vi "停止.vi"(1 "停止":bool) -> (0 "停止报文发送":string)   [LabVIEW 2023]
uses:
  <vilib>/Instr/_visa.llb/VISA Configure Serial Port (Instr).vi
panel:
  out "读取缓冲区":string
  out "返回数":u32
  in  "VISA resource name":refnum<visa-resource-name>="COM8" caption="VISA资源名称"
  out "错误输出":errorcluster
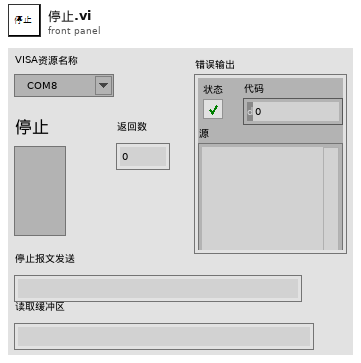
[diagram p1: front panel]
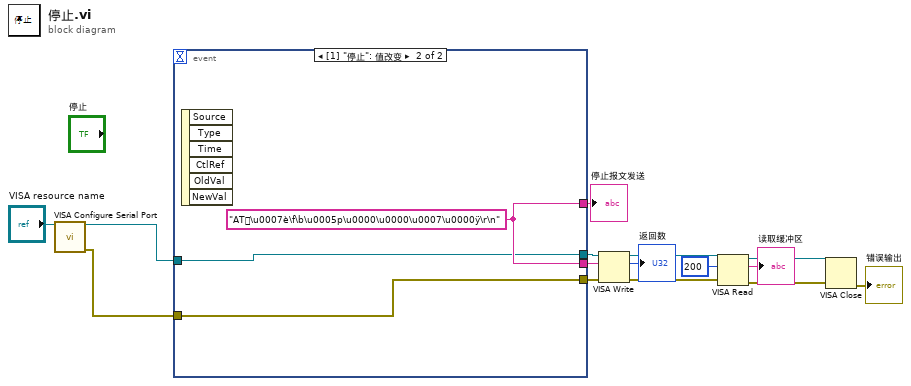
[diagram p0: block diagram]
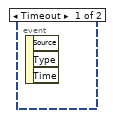
[diagram p2: hidden frame]
diagram:
  n1 = call-poly "VISA Configure Serial Port"("VISA resource name"="VISA resource name") -> ("VISA resource name out"=w6:refnum<visa-resource-name>, "error out"=w3:errorcluster)  [unwired: 13 in]
  n2 = event shown="[1] \"停止\": 值改变" {
    selector: _ -> [_ _]
    dyn-events: _ -> [_ _]
    timeout: _ -> [_ _]
    tunnel: [_ w18] -> w15
    tunnel: [_ w18] -> w7
    tunnel: w6 -> [_ w17]
    tunnel: [_ w17] -> w5
    tunnel: [_ w16] -> w4
    tunnel: w3 -> [_ w16]
    event Timeout {
      n3 = event-data() -> ()  [unwired: 1 in, 3 out]
    }
    event "停止": Value Change {
      w18 = "AT\u0007è\f\b\u0005p\u0000\u0000\u0007\u0000ÿ\r\n"
      n4 = event-data() -> ()  [unwired: 1 in, 6 out]
    }
  }
  "停止报文发送" <- w15
  n5 = VISA Write(VISA resource name=w5, write buffer=w7, error in (no error)=w4) -> (VISA resource name out=w14:refnum<visa-resource-name>, return count=→"返回数":u32, error out=w13:errorcluster)
  n6 = VISA Read(VISA resource name=w14, byte count=u32 200 ("字节总数"), error in (no error)=w13) -> (VISA resource name out=w12:refnum<visa-resource-name>, read buffer=→"读取缓冲区":string, error out=w11:errorcluster)  [unwired: 1 out]
  n7 = VISA Close(VISA resource name=w12, error in (no error)=w11) -> (error out=→"错误输出":errorcluster)
